vi "Read Multiple Attributes (Variant).vi"(4 "Value Type(s)":variant, 6 "error in (no error)":errorcluster, 8 "Names":string[](array[string]), 9 "HDF5 Ref":T1) -> (0 "error out":errorcluster, 1 "Value(s)":variant[](array[variant]), 2 "Names out":string[](array[string]), 3 "HDF5 Ref out":T1)   [LabVIEW 2017]
doc: "Reads multiple attributes attached to the specified HDF5 object. This VI is not meant to be called directly under most circumstances. Instead, call LVH5 Read Attributes.xnode [Read Attribute(s)].\n\nNote that the Value Type(s) input, if wired, should either be an array or a cluster. If a cluster is wired, the output will be an array of the member values."
uses:
  <vilib>/UPVI/lvhdf5/library.llb/HDF5 Ref.ctl
  <vilib>/Utility/VariantDataType/VariantType.lvlib
panel:
  # "LVHDF5 Toolkit\nCopyright (c) 2005-2013 by Jason D. Sommerville\nCopyright (c) 2014 by UPVI, LLC.\n\nThis use and distribution of this file is governed by the terms found in \nLICENSE.txt distributed with this toolkit and installed at\n <user.lib>\\_lvhdf5\\LICENSE.txt"
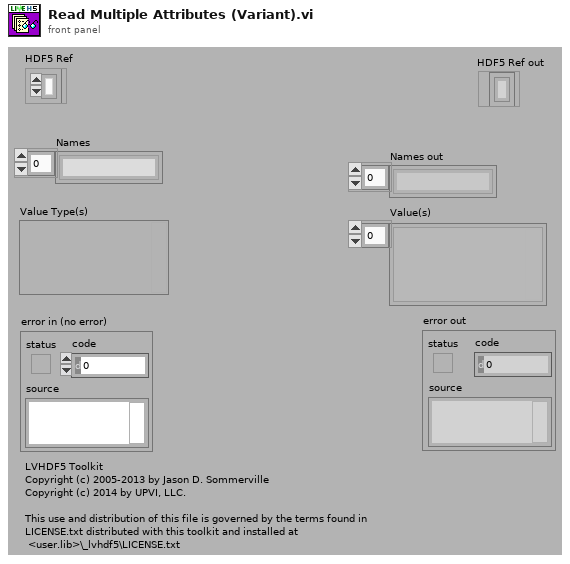
[diagram p1: front panel]
types:
  T1 = typedef "HDF5 Ref.ctl" = refnum<k1>
  T2 = typedef "VariantType.lvlib/Type.ctl" = enum8{"Invalid Type", "Void", "I8", "I16", "I32", "I64", "U8", "U16", "U32", "U64", "Single Float", "Double Float", "Extended Float", "Single Complex", "Double Complex", "Extended Complex", "Enum U8", "Enum U16", "Enum U32", "Enum U64", "Single Float With Unit", "Double Float With Unit", "Extended Float With Unit", "Single Complex with Unit", "Double Complex with Unit", "Extended Complex with Unit", "Boolean", "String", "Path", "Picture", "Tag", "Array", "Cluster", "Variant", "LV Variant", "Waveform", "Timestamp", "Digital Waveform", "Digital Data", "ExpressData", "Refnum", "External Data", "VI", "Poly VI", "LabVIEW Class Instance", "Fixed Point"}
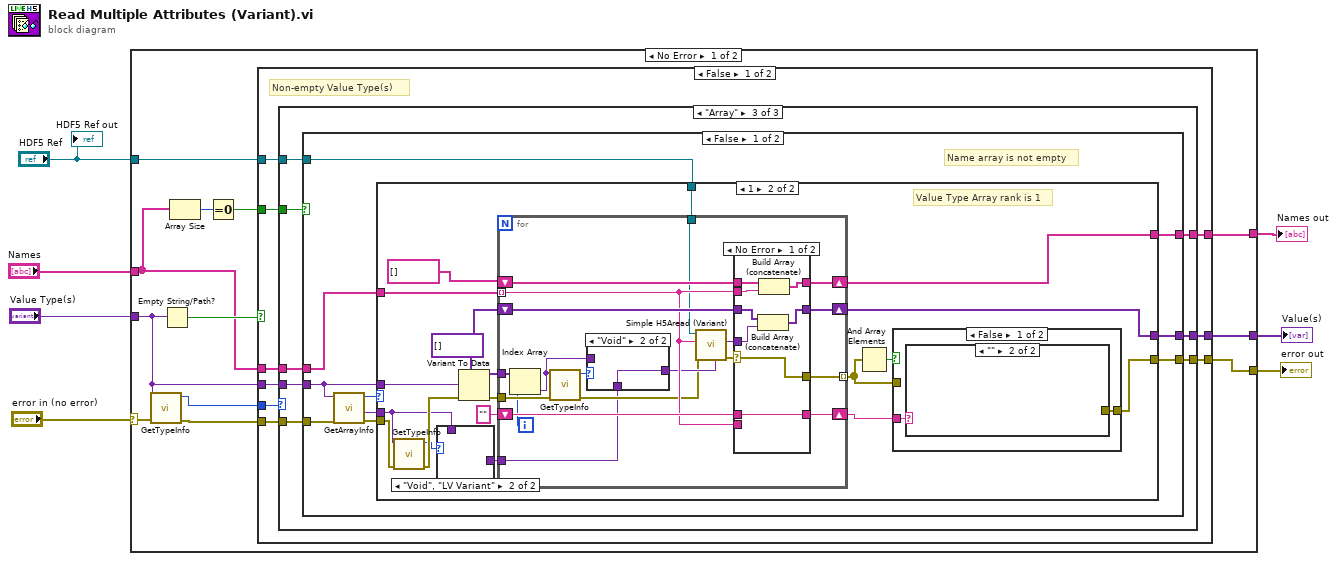
[diagram p0: block diagram]
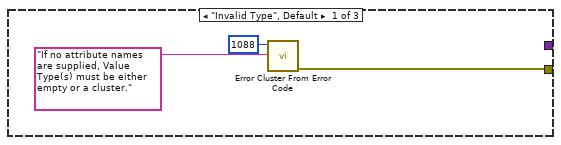
[diagram p2: hidden frame]
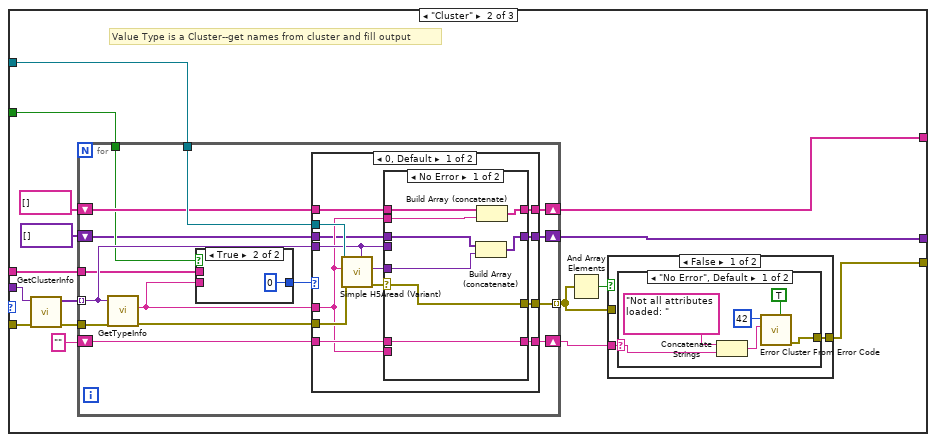
[diagram p3: hidden frame]
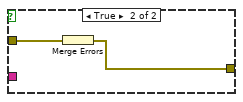
[diagram p5: hidden frame]
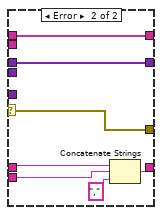
[diagram p6: hidden frame]
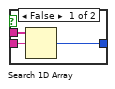
[diagram p8: hidden frame]
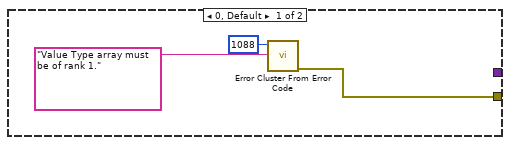
[diagram p9: hidden frame]
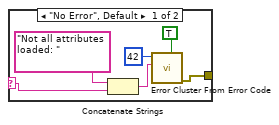
[diagram p11: hidden frame]
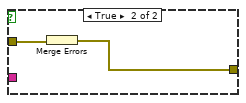
[diagram p12: hidden frame]
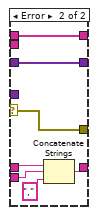
[diagram p14: hidden frame]
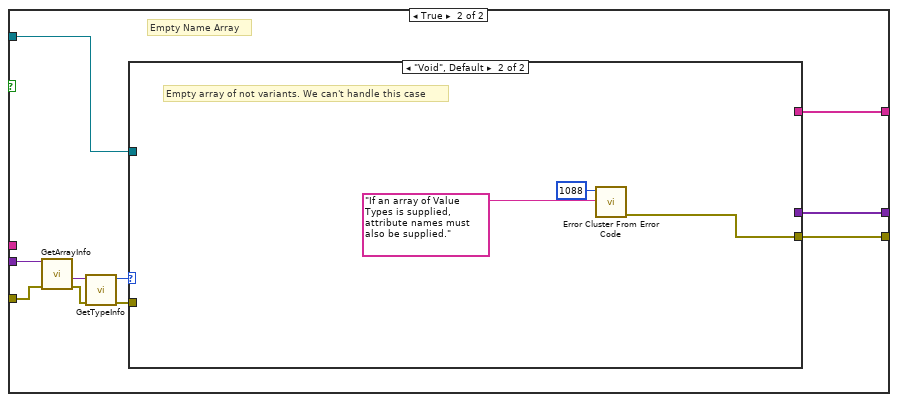
[diagram p15: hidden frame]
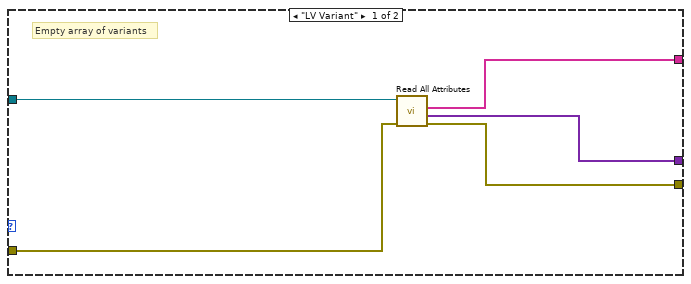
[diagram p16: hidden frame]
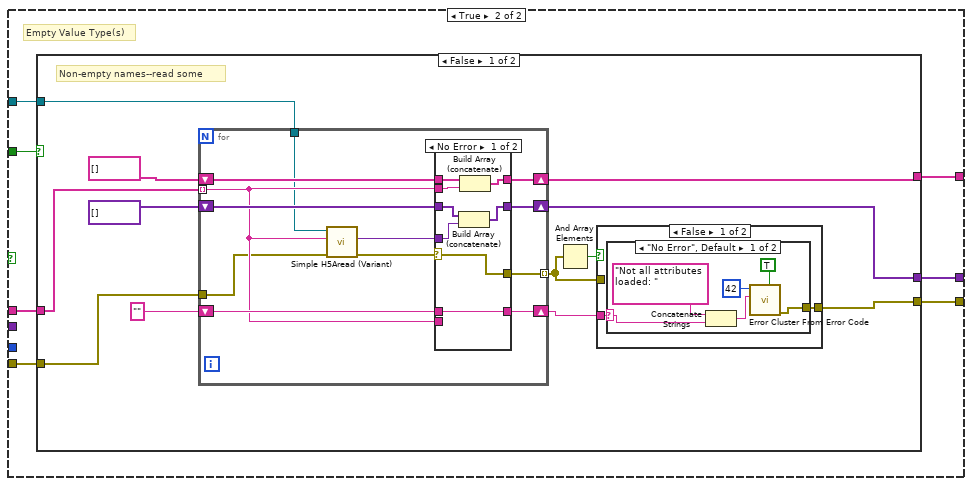
[diagram p17: hidden frame]
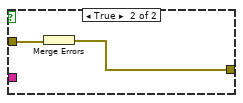
[diagram p19: hidden frame]
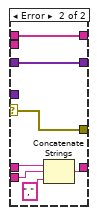
[diagram p20: hidden frame]
diagram:
  n1 = case shown="No Error" "error in (no error)" {
    selector: "error in (no error)" -> [w19 w275]
    tunnel: [w14 w275] -> w6
    tunnel: "HDF5 Ref" -> [w16 _]
    tunnel: [w12 string[] []] -> w4
    tunnel: [w15 variant[] []] -> w1
    tunnel: "Names" -> [w11 _]
    tunnel: "Value Type(s)" -> [w17 _]
    frame No Error {
      n2 = call <vilib>:"GetTypeInfo.vi"("error in (no error)"=w19, "Variant"=w17) -> ("error out"=w18:errorcluster, "Type Enum"=w8:T2)  [unwired: 5 in, 3 out]
      n3 = Empty String/Path?(string/path=w17) -> (empty?=w13:bool)
      n4 = Array Size(array=w11) -> (size(s)=w10:i32)
      n5 = Equal To 0?(x=w10) -> (x = 0?=w9:bool)
      n6 = case shown="False" w13 {
        tunnel: w8 -> [w28 _]
        tunnel: w18 -> [w27 w213]
        tunnel: w17 -> [w26 _]
        tunnel: w16 -> [w25 w219]
        tunnel: [w24 w217] -> w15
        tunnel: [w23 w216] -> w14
        tunnel: [w22 w218] -> w12
        tunnel: w11 -> [w21 w214]
        tunnel: w9 -> [w20 w215]
        frame False {
          # "Non-empty Value Type(s)"
          n7 = case shown="\"Array\"" w28 {
            tunnel: w27 -> [_ w47 w115]
            tunnel: w26 -> [_ w34 w114]
            tunnel: w25 -> [_ w44 w110]
            tunnel: [_ w32 w108] -> w24
            tunnel: [w29 w33 w112] -> w23
            tunnel: [_ w39 w109] -> w22
            tunnel: w21 -> [_ w38 w111]
            tunnel: w20 -> [_ w37 w113]
            frame "Invalid Type", Default {
              n8 = call <vilib>:"Error Cluster From Error Code.vi"("error message (\"\")"="If no attribute names are supplied, Value Type(s) must be either empty or a cluster." ("error message (\"\")"), "error code (0)"=1088) -> ("error out"=w29:errorcluster)  [unwired: 7 in]
            }
            frame "Cluster" {
              # "Value Type is a Cluster--get names from cluster and fill output"
              n9 = call <vilib>:"GetClusterInfo.vi"("error in (no error)"=w47, "Variant"=w34) -> ("error out"=w46:errorcluster, "Cluster Elements"=w45:variant[])  [unwired: 8 in]
              n10 = for {
                tunnel: w46 -> [w72]
                tunnel: w45 -> [w68] mode=indexing
                tunnel: w44 -> [w71]
                tunnel: [w69] -> w35 mode=indexing
                shift-right: [w67] -> w42
                shift-left: "" -> [w66]
                shift-right: [w64] -> w39
                shift-left: string[] [] ("Names") -> [w65]
                tunnel: w38 -> [w63]
                tunnel: w37 -> [w62]
                shift-right: [w59] -> w32
                shift-left: variant[] [] -> [w60]
                n11 = call <vilib>:"GetTypeInfo.vi"("error in (no error)"=w72, "Variant"=w68) -> ("error out"=w70:errorcluster, "Name"=w58:string)  [unwired: 5 in, 3 out]
                n12 = case shown="True" w62 {
                  tunnel: w58 -> [w106 _]
                  tunnel: w63 -> [w105 _]
                  tunnel: [w104 0 ("index of element")] -> w61
                  frame False {
                    n13 = Search 1D Array(1D array=w105, element=w106) -> (index of element=w104:i32)  [unwired: 1 in]
                  }
                  frame True {
                  }
                }
                n14 = case shown="0, Default" w61 {
                  tunnel: w71 -> [w85 _]
                  tunnel: w70 -> [w84 _]
                  tunnel: [w81 _] -> w69
                  tunnel: w68 -> [w80 _]
                  tunnel: [w79 w102] -> w67
                  tunnel: w66 -> [w78 w102]
                  tunnel: w65 -> [w77 w103]
                  tunnel: [w76 w103] -> w64
                  tunnel: w58 -> [w75 _]
                  tunnel: w60 -> [w74 w101]
                  tunnel: [w73 w101] -> w59
                  frame 0, Default {
                    n15 = call <vilib>:"Simple H5Aread (Variant).vi"("Type"=w80, "error in (no error)"=w84, "Name"=w75, "HDF5 Ref"=w85) -> ("error out"=w83:errorcluster, "Value"=w82:variant)  [unwired: 3 in, 1 out]
                    n16 = case shown="No Error" w83 {
                      selector: w83 -> [w87 w100]
                      tunnel: w82 -> [w86 _]
                      tunnel: [w87 w100] -> w81
                      tunnel: w80 -> [_ _]
                      tunnel: [w93 w98] -> w79
                      tunnel: w78 -> [w93 w99]
                      tunnel: w75 -> [_ w97]
                      tunnel: w77 -> [w92 w95]
                      tunnel: [w91 w95] -> w76
                      tunnel: w75 -> [w90 _]
                      tunnel: w74 -> [w89 w94]
                      tunnel: [w88 w94] -> w73
                      frame No Error {
                        n17 = Build Array (concatenate)(w89, w86) -> (w88:variant[])
                        n18 = Build Array (concatenate)(w92, w90) -> (w91:string[])
                      }
                      frame Error {
                        n19 = Concatenate Strings(w99, w97, "," ("string")) -> (w98:string)
                      }
                    }
                  }
                  frame -1 {
                    # "Skip this item"
                  }
                }
              }
              n20 = And Array Elements(Boolean array=w35) -> (logical AND=w41:bool)
              n21 = case shown="False" w41 {
                tunnel: w42 -> [w49 _]
                tunnel: [w48 w56] -> w33
                tunnel: w35 -> [_ w57]
                frame False {
                  n22 = case shown="\"No Error\", Default" w49 {
                    selector: w49 -> [w52 _]
                    tunnel: [w50 _] -> w48
                    frame "No Error", Default {
                      n23 = Concatenate Strings("Not all attributes loaded: " ("string"), w52) -> (w51:string)
                      n24 = call <vilib>:"Error Cluster From Error Code.vi"("is warning? (False)"=TRUE, "error message (\"\")"=w51, "error code (0)"=42) -> ("error out"=w50:errorcluster)  [unwired: 6 in]
                    }
                    frame "" {
                    }
                  }
                }
                frame True {
                  n25 = Merge Errors(w57) -> (w56:errorcluster)
                }
              }
            }
            frame "Array" {
              n26 = case shown="False" w113 {
                tunnel: w115 -> [w125 w202]
                tunnel: w114 -> [w120 w203]
                tunnel: [w123 w204] -> w112
                tunnel: w111 -> [w119 _]
                tunnel: w110 -> [w118 w197]
                tunnel: [w117 w196] -> w109
                tunnel: [w116 w195] -> w108
                frame False {
                  # "Name array is not empty"
                  n27 = call <vilib>:"GetArrayInfo.vi"("error in (no error)"=w125, "Variant"=w120) -> ("error out"=w121:errorcluster, "ArrayElement"=w122:variant, "NDims"=w124:i32)  [unwired: 6 in, 1 out]
                  n28 = case shown="1" w124 {
                    tunnel: [w126 w139] -> w123
                    tunnel: w122 -> [_ w130]
                    tunnel: w121 -> [_ w133]
                    tunnel: w120 -> [_ w147]
                    tunnel: w119 -> [_ w144]
                    tunnel: w118 -> [_ w143]
                    tunnel: [_ w140] -> w117
                    tunnel: [_ w134] -> w116
                    frame 0, Default {
                      n29 = call <vilib>:"Error Cluster From Error Code.vi"("error message (\"\")"="Value Type array must be of rank 1." ("error message (\"\")"), "error code (0)"=1088) -> ("error out"=w126:errorcluster)  [unwired: 7 in]
                    }
                    frame 1 {
                      w146 = variant[] []
                      # "Value Type Array rank is 1"
                      n30 = call <vilib>:"GetTypeInfo.vi"("error in (no error)"=w133, "Variant"=w130) -> ("error out"=w132:errorcluster, "Type Enum"=w131:T2)  [unwired: 5 in, 3 out]
                      n31 = case shown="\"Void\", \"LV Variant\"" w131 {
                        tunnel: w130 -> [w148 _]
                        tunnel: [w148 _] -> w129
                        frame "Invalid Type", Default {
                        }
                        frame "Void", "LV Variant" {
                        }
                      }
                      n32 = Variant To Data(error in=w132, type=w146, Variant=w147) -> (data=w145:variant[], error out=w138:errorcluster)
                      n33 = for {
                        tunnel: w145 -> [w161]
                        tunnel: [w177] -> w135 mode=indexing
                        shift-right: [w176] -> w136
                        shift-left: "" -> [w175]
                        shift-right: [w173] -> w140
                        shift-left: string[] [] -> [w174]
                        shift-right: [w171] -> w134
                        shift-left: w146 -> [w172]
                        tunnel: w144 -> [w168] mode=indexing
                        tunnel: w143 -> [w167]
                        tunnel: w138 -> [w166]
                        tunnel: w129 -> [w159]
                        i -> [w162]
                        n34 = Index Array(array=w161, index=w162) -> (element=w160:variant)
                        n35 = call <vilib>:"GetTypeInfo.vi"("error in (no error)"=w166, "Variant"=w160) -> ("error out"=w163:errorcluster, "Type Enum"=w165:T2)  [unwired: 5 in, 3 out]
                        n36 = case shown="\"Void\"" w165 {
                          tunnel: w160 -> [w178 _]
                          tunnel: w159 -> [_ w179]
                          tunnel: [w178 w179] -> w164
                          frame "I32", Default {
                          }
                          frame "Void" {
                          }
                        }
                        n37 = call <vilib>:"Simple H5Aread (Variant).vi"("Type"=w164, "error in (no error)"=w163, "Name"=w168, "HDF5 Ref"=w167) -> ("error out"=w170:errorcluster, "Value"=w169:variant)  [unwired: 3 in, 1 out]
                        n38 = case shown="No Error" w170 {
                          selector: w170 -> [w187 w194]
                          tunnel: w169 -> [w182 _]
                          tunnel: [w187 w194] -> w177
                          tunnel: [w186 w192] -> w176
                          tunnel: w175 -> [w186 w193]
                          tunnel: w168 -> [_ w191]
                          tunnel: w174 -> [w185 w189]
                          tunnel: [w184 w189] -> w173
                          tunnel: w168 -> [w183 _]
                          tunnel: w172 -> [w181 w188]
                          tunnel: [w180 w188] -> w171
                          frame No Error {
                            n39 = Build Array (concatenate)(w181, w182) -> (w180:variant[])
                            n40 = Build Array (concatenate)(w185, w183) -> (w184:string[])
                          }
                          frame Error {
                            n41 = Concatenate Strings(w193, w191, "," ("string")) -> (w192:string)
                          }
                        }
                      }
                      n42 = And Array Elements(Boolean array=w135) -> (logical AND=w142:bool)
                      n43 = case shown="False" w142 {
                        tunnel: [w150 w157] -> w139
                        tunnel: w135 -> [_ w158]
                        tunnel: w136 -> [w149 _]
                        frame False {
                          n44 = case shown="\"\"" w149 {
                            selector: w149 -> [w153 _]
                            tunnel: [w151 _] -> w150
                            frame "No Error", Default {
                              n45 = Concatenate Strings("Not all attributes loaded: " ("string"), w153) -> (w152:string)
                              n46 = call <vilib>:"Error Cluster From Error Code.vi"("is warning? (False)"=TRUE, "error message (\"\")"=w152, "error code (0)"=42) -> ("error out"=w151:errorcluster)  [unwired: 6 in]
                            }
                            frame "" {
                            }
                          }
                        }
                        frame True {
                          n47 = Merge Errors(w158) -> (w157:errorcluster)
                        }
                      }
                    }
                  }
                }
                frame True {
                  # "Empty Name Array"
                  n48 = call <vilib>:"GetArrayInfo.vi"("error in (no error)"=w202, "Variant"=w203) -> ("error out"=w200:errorcluster, "ArrayElement"=w201:variant)  [unwired: 6 in, 2 out]
                  n49 = call <vilib>:"GetTypeInfo.vi"("error in (no error)"=w200, "Variant"=w201) -> ("error out"=w198:errorcluster, "Type Enum"=w199:T2)  [unwired: 5 in, 3 out]
                  n50 = case shown="\"Void\", Default" w199 {
                    tunnel: [w207 w210] -> w204
                    tunnel: w198 -> [w208 _]
                    tunnel: w197 -> [w209 _]
                    tunnel: [w206 _] -> w196
                    tunnel: [w205 _] -> w195
                    frame "LV Variant" {
                      # "Empty array of variants"
                      n51 = call <vilib>:"Read All Attributes.vi"("error in (no error)"=w208, "HDF5 Ref"=w209) -> ("error out"=w207:errorcluster, "Values"=w205:variant[], "Names"=w206:string[])  [unwired: 4 in, 1 out]
                    }
                    frame "Void", Default {
                      # "Empty array of not variants. We can't handle this case"
                      n52 = call <vilib>:"Error Cluster From Error Code.vi"("error message (\"\")"="If an array of Value Types is supplied, attribute names must also be supplied." ("error message (\"\")"), "error code (0)"=1088) -> ("error out"=w210:errorcluster)  [unwired: 7 in]
                    }
                  }
                }
              }
            }
          }
        }
        frame True {
          # "Empty Value Type(s)"
          n53 = case shown="False" w215 {
            tunnel: w219 -> [w221 w272]
            tunnel: [w222 w271] -> w218
            tunnel: [w220 w270] -> w217
            tunnel: [w223 w269] -> w216
            tunnel: w214 -> [w225 _]
            tunnel: w213 -> [w224 _]
            frame False {
              # "Non-empty names--read some"
              n54 = for {
                tunnel: [w253] -> w226 mode=indexing
                shift-right: [w252] -> w227
                shift-left: "" -> [w251]
                shift-right: [w249] -> w222
                shift-left: string[] [] -> [w250]
                shift-right: [w247] -> w220
                shift-left: variant[] [] -> [w248]
                tunnel: w225 -> [w244] mode=indexing
                tunnel: w224 -> [w243]
                tunnel: w221 -> [w242]
                n55 = call <vilib>:"Simple H5Aread (Variant).vi"("error in (no error)"=w243, "Name"=w244, "HDF5 Ref"=w242) -> ("error out"=w246:errorcluster, "Value"=w245:variant)  [unwired: 4 in, 1 out]
                n56 = case shown="No Error" w246 {
                  selector: w246 -> [w261 w268]
                  tunnel: w245 -> [w256 _]
                  tunnel: [w261 w268] -> w253
                  tunnel: [w260 w266] -> w252
                  tunnel: w251 -> [w260 w267]
                  tunnel: w244 -> [_ w265]
                  tunnel: w250 -> [w259 w263]
                  tunnel: [w258 w263] -> w249
                  tunnel: w244 -> [w257 _]
                  tunnel: w248 -> [w255 w262]
                  tunnel: [w254 w262] -> w247
                  frame No Error {
                    n57 = Build Array (concatenate)(w255, w256) -> (w254:variant[])
                    n58 = Build Array (concatenate)(w259, w257) -> (w258:string[])
                  }
                  frame Error {
                    n59 = Concatenate Strings(w267, w265, "," ("string")) -> (w266:string)
                  }
                }
              }
              n60 = And Array Elements(Boolean array=w226) -> (logical AND=w230:bool)
              n61 = case shown="False" w230 {
                tunnel: [w233 w240] -> w223
                tunnel: w226 -> [_ w241]
                tunnel: w227 -> [w232 _]
                frame False {
                  n62 = case shown="\"No Error\", Default" w232 {
                    selector: w232 -> [w236 _]
                    tunnel: [w234 _] -> w233
                    frame "No Error", Default {
                      n63 = Concatenate Strings("Not all attributes loaded: " ("string"), w236) -> (w235:string)
                      n64 = call <vilib>:"Error Cluster From Error Code.vi"("is warning? (False)"=TRUE, "error message (\"\")"=w235, "error code (0)"=42) -> ("error out"=w234:errorcluster)  [unwired: 6 in]
                    }
                    frame "" {
                    }
                  }
                }
                frame True {
                  n65 = Merge Errors(w241) -> (w240:errorcluster)
                }
              }
            }
            frame True {
              # "Empty Names - Read All"
              n66 = call <vilib>:"Read All Attributes.vi"("HDF5 Ref"=w272) -> ("error out"=w269:errorcluster, "Values"=w270:variant[], "Names"=w271:string[])  [unwired: 5 in, 1 out]
            }
          }
        }
      }
    }
    frame Error {
    }
  }
  "error out" <- w6
  "Names out" <- w4
  "Value(s)" <- w1
  "HDF5 Ref out" <- "HDF5 Ref"
